vi "Increment_Run_Time.vi"(7 "error in (no error)":errorcluster, 10 "Data Cluster in":T1) -> (0 "error out":errorcluster, 2 "Increment Run Time?":bool, 3 "Data Cluster out":T1)   [LabVIEW 2026]
uses:
  controls/UI Data.ctl
  controls/Display_Panel.ctl
  controls/Controls.ctl
  controls/Program_Settings.ctl
panel:
  # "Manual Setting"
  # "Manual Setting"
  # "Manual Setting"
  # "Manual Setting"
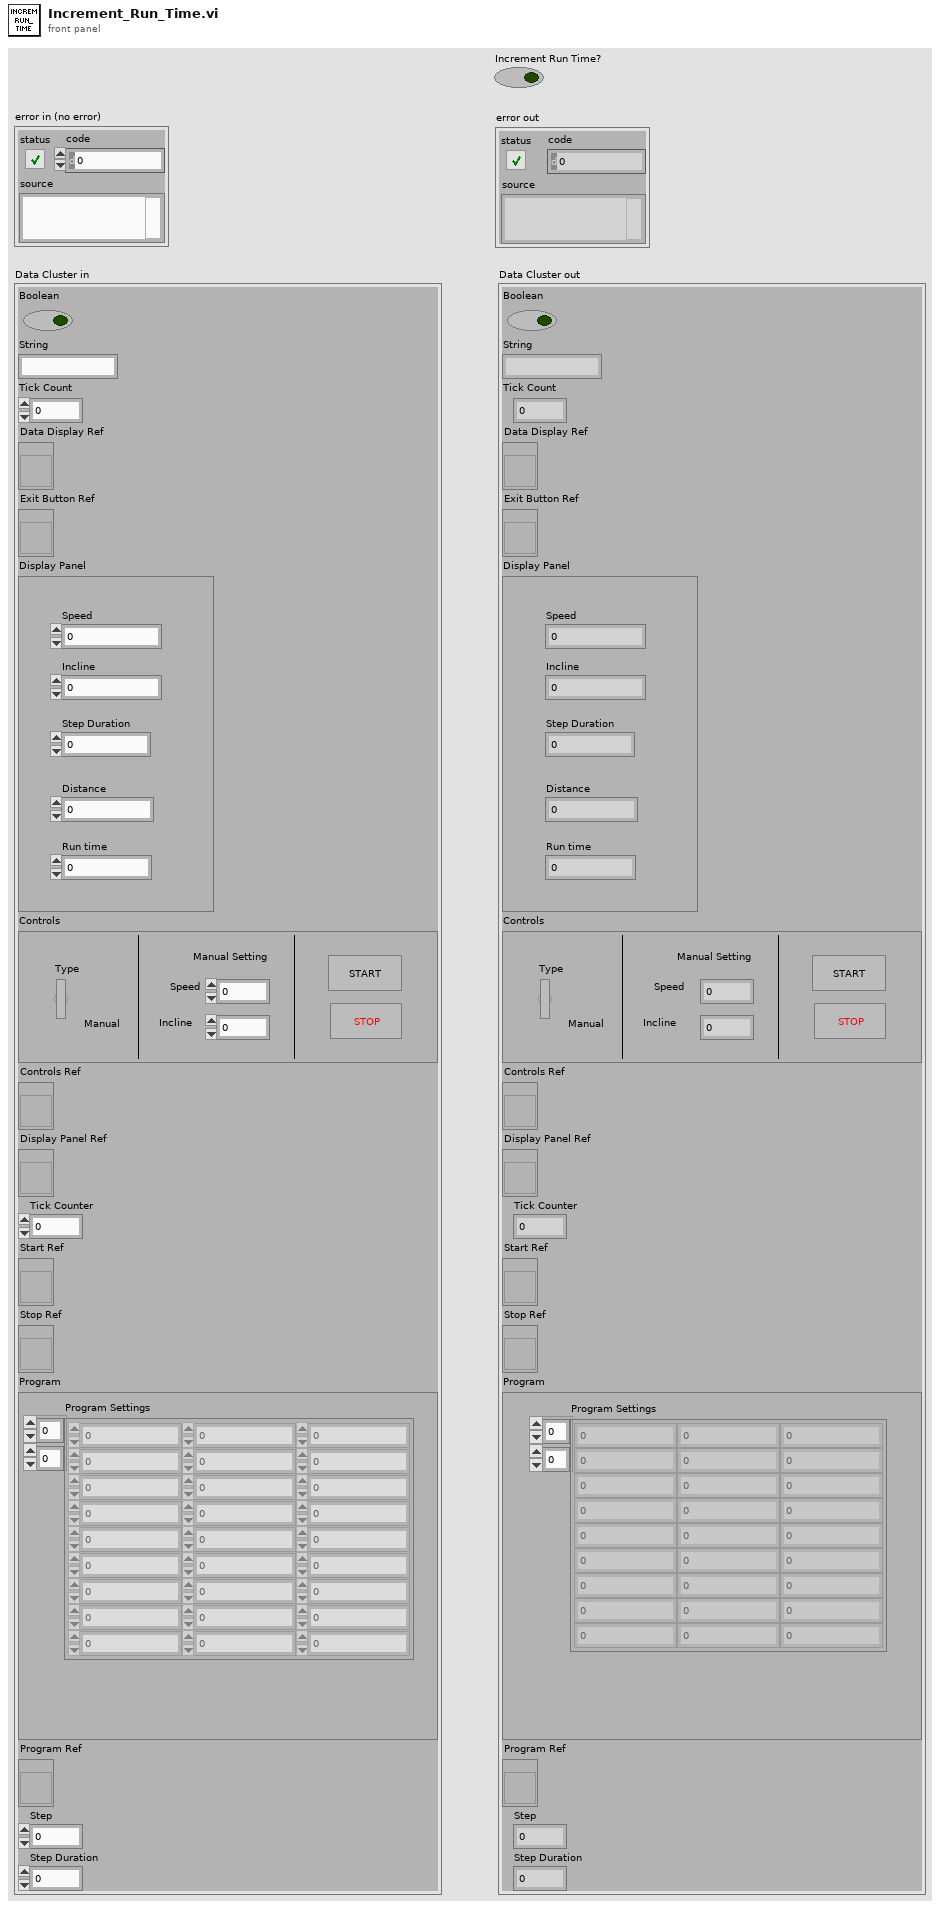
[diagram p1: front panel]
types:
  T1 = typedef "UI Data.ctl" = cluster{"Boolean":bool, "String":string, "Tick Count":dbl, "Data Display Ref":refnum<vi>, "Exit Button Ref":refnum<vi>, "Display Panel":T2, "Controls":T3, "Controls Ref":refnum<vi>, "Display Panel Ref":refnum<vi>, "Tick Counter":dbl, "Start Ref":refnum<vi>, "Stop Ref":refnum<vi>, "Program":T4, "Program Ref":refnum<vi>, "Step":u32, "Step Duration":dbl}
  T2 = typedef "Display_Panel.ctl" = cluster{"Speed":dbl, "Incline":dbl, "Step Duration":dbl, "Distance":dbl, "Run time":dbl}
  T3 = typedef "Controls.ctl" = cluster{"Type":bool, "Speed":dbl, "Incline":dbl, "Start":bool, "stop":bool}
  T4 = typedef "Program_Settings.ctl" = cluster{"Program Settings":dbl[][]}
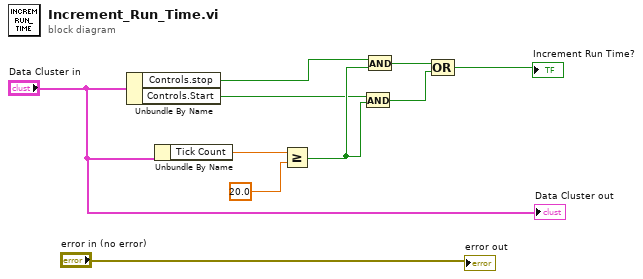
[diagram p0: block diagram]
diagram:
  n1 = Unbundle By Name("Data Cluster in") -> ("Controls.stop"=w5:bool, "Controls.Start"=w4:bool)
  n2 = Unbundle By Name("Data Cluster in") -> ("Tick Count"=w8:dbl)
  n3 = Greater Or Equal?(x=w8, y=20.0) -> (x >= y?=w7:bool)
  n4 = And(x=w4, y=w7) -> (x .and. y?=w2:bool)
  n5 = And(x=w5, y=w7) -> (x .and. y?=w3:bool)
  n6 = Compound Arithmetic op=OR(w3, w2) -> (→"Increment Run Time?":bool)
  "error out" <- "error in (no error)"
  "Data Cluster out" <- "Data Cluster in"
